vi "Load Parameter.vi"(8 "error in (no error)":errorcluster, 10 "Resource":variant, 11 "Analyze BaseClass in":refnum<class "Analyze BaseClass.lvclass">) -> (0 "error out":errorcluster, 3 "Analyze BaseClass out":refnum<class "Analyze BaseClass.lvclass">)   [LabVIEW 2014, in "Analyze.lvlib" / "Analyze BaseClass.lvlib" / "Analyze BaseClass.lvclass"]
uses:
  Analyze BaseClass.lvclass
  Analyze Parameter/Analyze Parameter Base/Analyze Parameter Base.lvclass
  Analyze BaseClass.lvclass/Analyze BaseClass.ctl
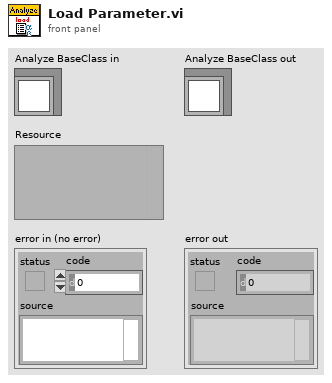
[diagram p1: front panel]
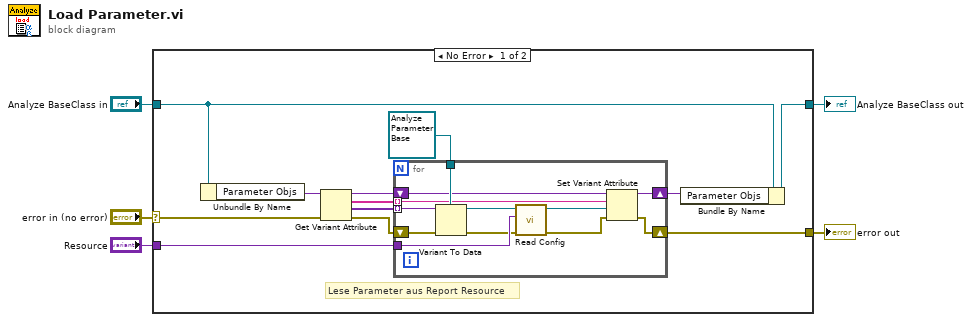
[diagram p0: block diagram]
diagram:
  n1 = case shown="No Error" "error in (no error)" {
    selector: "error in (no error)" -> [w9 w31]
    tunnel: [w8 w31] -> w4
    tunnel: [w7 w30] -> w2
    tunnel: "Analyze BaseClass in" -> [w17 w30]
    tunnel: "Resource" -> [w11 _]
    frame No Error {
      # "Lese Parameter aus Report Resource"
      n2 = Unbundle By Name(w17) -> ("Parameter Objs"=w16:variant)
      n3 = Get Variant Attribute(Variant=w16, error in=w9) -> (duplicate Variant=w13:variant, names=w10:string[], values=w14:variant[], error out=w12:errorcluster)  [unwired: 2 in]
      n4 = for {
        tunnel: refnum<class "Analyze Parameter Base.lvclass"> refnum ("Analyze Parameter Base.lvclass") -> [w29]
        tunnel: w14 -> [w28] mode=indexing
        shift-right: [w22] -> w6
        shift-left: w13 -> [w21]
        shift-right: [w23] -> w8
        shift-left: w12 -> [w27]
        tunnel: w11 -> [w25]
        tunnel: w10 -> [w20] mode=indexing
        n5 = Variant To Data(error in=w27, type=w29, Variant=w28) -> (data=w26:refnum<class "Analyze Parameter Base.lvclass">, error out=w24:errorcluster)
        n6 = call-dynamic "Read Config.vi"("error in (no error)"=w24, "Resource In"=w25, "Analyze Parameter Base in"=w26) -> ("error out"=w18:errorcluster, "Analyze Parameter Base out"=w19:refnum<class "Analyze Parameter Base.lvclass">)  [unwired: 6 in, 1 out]
        n7 = Set Variant Attribute(Variant=w21, name=w20, value=w19, error in=w18) -> (Variant out=w22:variant, error out=w23:errorcluster)  [unwired: 1 out]
      }
      n8 = Bundle By Name(cluster=w17, "Parameter Objs"=w6) -> (w7:refnum<class "Analyze BaseClass.lvclass">)
    }
    frame Error {
    }
  }
  "error out" <- w4
  "Analyze BaseClass out" <- w2
